vi "Test.vi"   [LabVIEW 2012]
doc: "This VI is called when test mode begins, and will automatically be terminated when it ends. You can add manual or automatic tests and invoke them from the dashboard."
uses:
  Robot Global Data.vi
  <vilib>/Rock Robotics/WPI/RobotDrive/WPI_RobotDriveGetSetRefNum.vi
types:
  T1 = typedef "WPI_RobotDriveDevRef.ctl" = cluster{"DevStatus":errorcluster, "Motors[]":T2[], "Square Inputs":bool, "Max Output":dbl, "Isochronous":bool}
  T2 = typedef "WPI_MotorControlDeviceRef.ctl" = cluster{"DeviceStatus":errorcluster, "Type":enum16{"PWM", "CAN"}, "PWM":cluster{"Digital Module":T3, "PWM Channel":T4, "DeadBand":T5}, "CAN":cluster{"Device Number":u8, "Control Mode":T6, "Semaphore":T7, "Max Vout":dbl}, "Invert":bool, "TransformRef":T8, "InvTransformRef":T8}
  T3 = typedef "FPGA_TypedefDigitalModule.ctl" = enum16{"Digital Module 1", "Digital Module 2"}
  T4 = typedef "FPGA_DIOPWMChannel.ctl" = enum8{"PWM 1", "PWM 2", "PWM 3", "PWM 4", "PWM 5", "PWM 6", "PWM 7", "PWM 8", "PWM 9", "PWM 10", "Invalid"}
  T5 = typedef "WPI_PWMDeadband.ctl" = cluster{"Name":string, "maxPositivePwm":i32, "minPositivePwm":i32, "centerPwm":i32, "maxNegativePwm":i32, "minNegativePwm":i32, "angularRange":u16}
  T6 = typedef "WPI_CANJaguar_ControlMode.ctl" = enum8{"Percent VBus", "Current", "Speed", "Position", "Voltage"}
  T7 = typedef "Semaphore RefNum" = refnum<k1>
  T8 = typedef "WPI_PWMTransform_ConPane.ctl" = refnum<vi>
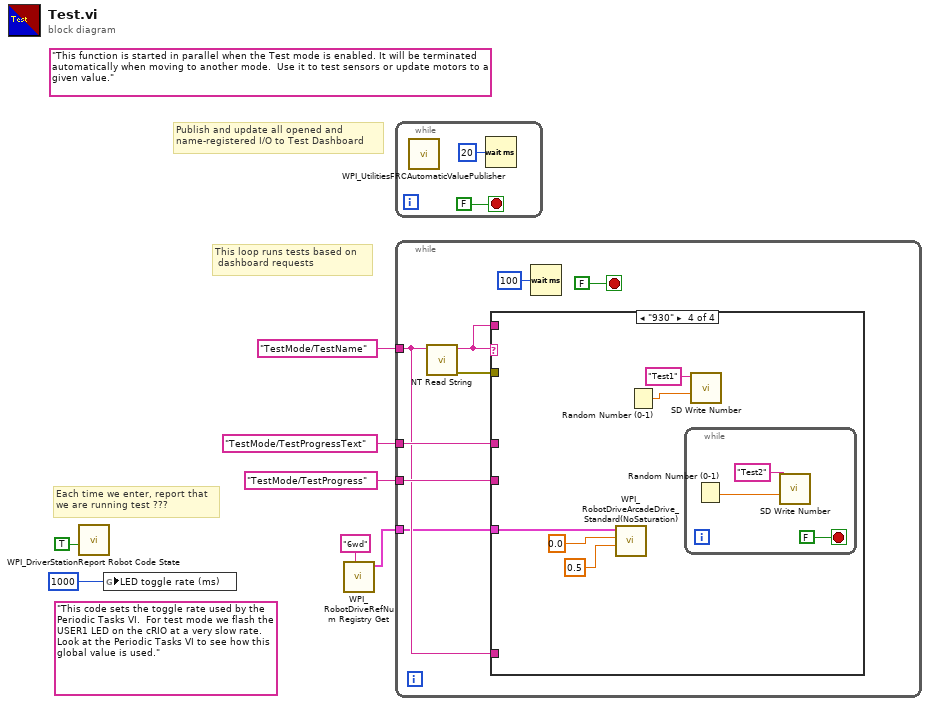
[diagram p0: block diagram]
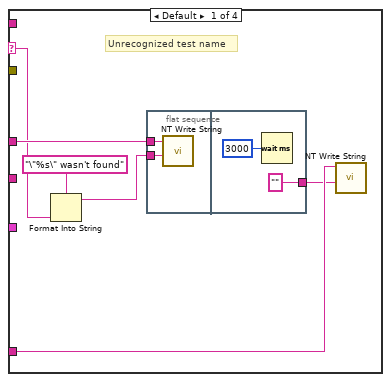
[diagram p2: hidden frame]
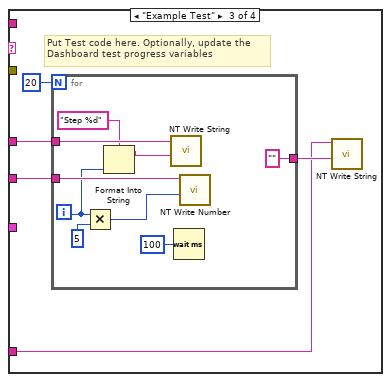
[diagram p4: hidden frame]
diagram:
  (unwired) "This code sets the toggle rate used by the Periodic Tasks VI.  For test mode we flash the USER1 LED on the cRIO at a very slow rate.  Look at the Periodic Tasks VI to see how this global value is used."
  (unwired) "This function is started in parallel when the Test mode is enabled. It will be terminated automatically when moving to another mode.  Use it to test sensors or update motors to a given value."
  # "This loop runs tests based on \n dashboard requests"
  # "Publish and update all opened and\nname-registered I/O to Test Dashboard"
  # "Each time we enter, report that\nwe are running test ???"
  n1 = call <vilib>:"WPI_DriverStationReport Robot Code State.vi"("TeleOp"=TRUE ("Autonomous")) -> ()  [unwired: 10 in, 1 out]
  n2 = global write "Robot Global Data.vi" "LED toggle rate (ms)"(u32 1000 ("LED ms toggle rate")) -> ()
  n3 = call <vilib>:"WPI_RobotDriveRefNum Registry Get.vi"("refnum name"="6wd") -> ("RobotDriveDevRef"=w1:T1)  [unwired: 1 in, 9 out]
  n4 = while {
    stop <- FALSE stop-if-true
    n5 = call <vilib>:"WPI_UtilitiesFRCAutomaticValuePublisher.vi"() -> ()  [unwired: 12 in]
    n6 = Wait (ms)(milliseconds to wait=u32 20) -> ()  [unwired: 1 out]
  }
  n7 = while {
    tunnel: "TestMode/TestName" ("Name") -> [w12]
    tunnel: "TestMode/TestProgressText" ("Name") -> [w15]
    tunnel: "TestMode/TestProgress" ("Name") -> [w14]
    tunnel: w1 -> [w10]
    stop <- FALSE stop-if-true
    n8 = call <vilib>:"NT Read String.vi"("Name"=w12) -> ("error out"=w11:errorcluster, "String"=w13:string)  [unwired: 9 in]
    n9 = case shown="\"930\"" w13 {
      selector: w13 -> [w22 _ _ _]
      tunnel: w12 -> [w19 _ w28 _]
      tunnel: w15 -> [w23 _ w31 _]
      tunnel: w14 -> [_ _ w32 _]
      tunnel: w13 -> [_ _ _ _]
      tunnel: w11 -> [_ _ _ _]
      tunnel: w10 -> [_ _ _ w46]
      frame Default {
        # "Unrecognized test name"
        n10 = Format Into String(format string="\"%s\" wasn't found" ("Name"), w22) -> (resulting string=w21:string)  [unwired: 2 in, 1 out]
        n11 = flat-sequence {
          tunnel: w23 -> [w24]
          tunnel: w21 -> [w25]
          tunnel: ["" ("Name")] -> w18
          frame #0 {
            n12 = call <vilib>:"NT Write String.vi"("String"=w25, "Name"=w24) -> ()  [unwired: 9 in, 1 out]
          }
          frame #1 {
            n13 = Wait (ms)(milliseconds to wait=u32 3000) -> ()  [unwired: 1 out]
          }
        }
        n14 = call <vilib>:"NT Write String.vi"("String"=w18, "Name"=w19) -> ()  [unwired: 9 in, 1 out]
      }
      frame "" {
        # "No test to run"
      }
      frame "Example Test" {
        # "Put Test code here. Optionally, update the\nDashboard test progress variables"
        n15 = for {
          N: 20 -> [_]
          tunnel: w32 -> [w41]
          tunnel: w31 -> [w39]
          tunnel: ["" ("String")] -> w29
          i -> [w36]
          n16 = Multiply(x=w36, y=u32 5 ("milliseconds to wait")) -> (x*y=w37:u32)
          n17 = Format Into String(format string="Step %d", w36) -> (resulting string=w34:string)  [unwired: 2 in, 1 out]
          n18 = call <vilib>:"NT Write String.vi"("String"=w34, "Name"=w39) -> ()  [unwired: 9 in, 1 out]
          n19 = Wait (ms)(milliseconds to wait=u32 100) -> ()  [unwired: 1 out]
          n20 = call <vilib>:"NT Write Number.vi"("Numeric"=w37, "Name"=w41) -> ()  [unwired: 9 in, 1 out]
        }
        n21 = call <vilib>:"NT Write String.vi"("String"=w29, "Name"=w28) -> ()  [unwired: 9 in, 1 out]
      }
      frame "930" {
        n22 = call <vilib>:"WPI_RobotDriveArcadeDrive_Standard(NoSaturation).vi"("Y axis value"=0.5, "X axis value"=0.0, "RobotDriveDevRef"=w46) -> ()  [unwired: 1 in, 8 out]
        n23 = Random Number (0-1)() -> (number: 0 to 1=w43:dbl)
        n24 = while {
          stop <- FALSE stop-if-true
          n25 = Random Number (0-1)() -> (number: 0 to 1=w48:dbl)
          n26 = call <vilib>:"SD Write Number.vi"("Numeric"=w48, "Name"="Test2") -> ()  [unwired: 8 in, 2 out]
        }
        n27 = call <vilib>:"SD Write Number.vi"("Numeric"=w43, "Name"="Test1") -> ()  [unwired: 8 in, 2 out]
      }
    }
    n28 = Wait (ms)(milliseconds to wait=u32 100) -> ()  [unwired: 1 out]
  }
